vi "GetType.vi"(8 "error in (no error)":errorcluster, 11 "Configure Frequency Voltage Range [FVR] Msg":refnum<class "Configure Frequency Voltage Range [FVR] Msg.lvclass">) -> (0 "error out":errorcluster, 2 "Data Sample":variant, 3 "Configure Frequency Voltage Range [FVR] Msg":refnum<class "Configure Frequency Voltage Range [FVR] Msg.lvclass">)   [LabVIEW 2015, in "CS++DMM.lvlib" / "Configure Frequency Voltage Range [FVR] Msg.lvclass"]
uses:
  Configure Frequency Voltage Range [FVR] Msg.lvclass
  Configure Frequency Voltage Range [FVR] Msg.lvclass/Configure Frequency Voltage Range [FVR] Msg.ctl
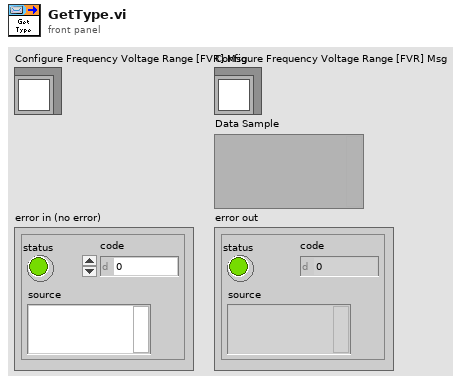
[diagram p1: front panel]
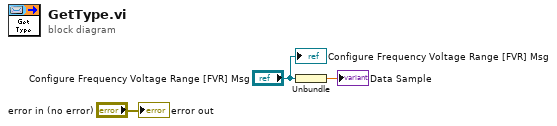
[diagram p0: block diagram]
diagram:
  n1 = Unbundle("Configure Frequency Voltage Range [FVR] Msg") -> (→"Data Sample":dbl)
  "error out" <- "error in (no error)"
  "Configure Frequency Voltage Range [FVR] Msg" <- "Configure Frequency Voltage Range [FVR] Msg"
